vi "GetOperationCycleId.vi"(8 "error in":errorcluster, 11 "OperationCycle in":refnum<class "OperationCycle.lvclass">) -> (0 "error out":errorcluster, 2 "OperationCycleId":string, 3 "OperationCycle out":refnum<class "OperationCycle.lvclass">)   [LabVIEW 2021, in "ProligentXMLGenerator.lvlib" / "OperationCycle.lvclass"]
doc: "Defines an ID for this operation cycle. This ID should be reused when providing results for an operation cycle spanned over multiple files. \n If no OperationCycleId is provided, all the results of this operation cycle must be provided in the context of a single OperationCycle.\nThe OperationCycleId must be unique across process runs."
uses:
  OperationCycle.lvclass
  OperationCycle.lvclass/OperationCycle.ctl
  Base/Attribute/Attribute.lvclass
  Base/Guid/Guid.lvclass
  C:/Projects/proligent-xml-generator-labview/src/ProligentXMLGenerator/Base/NonEmptyString/NonEmptyString.lvclass
  C:/Projects/proligent-xml-generator-labview/src/ProligentXMLGenerator/Base/String/String.lvclass
  C:/Projects/proligent-xml-generator-labview/src/ProligentXMLGenerator/Base/Attribute/Attribute.lvclass
  C:/Projects/proligent-xml-generator-labview/src/ProligentXMLGenerator/Base/Guid/Guid.lvclass
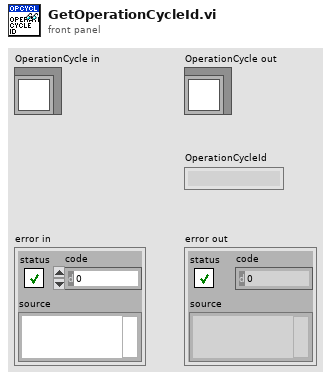
[diagram p1: front panel]
types:
  T1 = typedef "ProligentXMLGenerator.lvlib/OperationCycle.lvclass/Data.ctl" = cluster{"Name":string, "CustomData":refnum<class "CustomData.lvclass">, "ProcessFullName":refnum<class "ProcessFullName.lvclass">, "ProcessVersion":refnum<class "NonEmptyString_64.lvclass">, "OperationCycleId":refnum<class "Guid.lvclass">, "OperationName":refnum<class "NonEmptyString_65.lvclass">, "Location":refnum<class "FullName.lvclass">, "User":refnum<class "NonEmptyString_255.lvclass">, "OperationCycleStatus":refnum<class "ExecutionStatus.lvclass">, "OperationCycleStartTime":refnum<class "DateTime.lvclass">, "OperationCycleEndTime":refnum<class "DateTime.lvclass">, "TimeZoneInfoId":string}
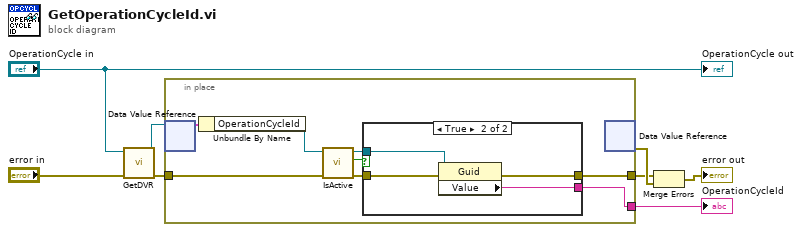
[diagram p0: block diagram]
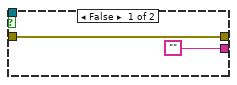
[diagram p2: hidden frame]
diagram:
  n1 = call "GetDVR.vi"("error in"="error in", "OperationCycle in"="OperationCycle in") -> ("error out"=w3:errorcluster, "DVRReference"=w2:refnum<data-value>)  [unwired: 8 in]
  n2 = in-place "In Place Element Structure" {
    in-place-border: [w15] -> w7
    in-place-border: w3 -> [w12]
    in-place-border: [w14] -> w5
    n3 = in-place-dvr #1(w2) -> (w16:T1)  [unwired: 1 out]
    n4 = Unbundle By Name(w16) -> ("OperationCycleId"=w11:refnum<class "Guid.lvclass">)
    n5 = call "IsActive.vi"("error in"=w12, "Attribute in"=w11) -> ("error out"=w13:errorcluster, "IsActive"=w9:bool, "Attribute in"=w10:refnum<class "Guid.lvclass">)  [unwired: 7 in]
    n6 = case shown="True" w9 {
      tunnel: ["" ("Empty String Constant") w22] -> w15
      tunnel: [w17 w21] -> w14
      tunnel: w13 -> [w17 w20]
      tunnel: w10 -> [_ w19]
      frame False {
      }
      frame True {
        n7 = property on="Property Node" class="Guid"(reference=w19, error in=w20) -> (error out=w21:errorcluster, "Value"=w22:string)  [unwired: 1 out]
      }
    }
    n8 = in-place-dvr #1() -> (w8:errorcluster)  [unwired: 1 in, 1 out]
  }
  "OperationCycleId" <- w7
  n9 = Merge Errors(w5, w8) -> (→"error out":errorcluster)
  "OperationCycle out" <- "OperationCycle in"
